vi "DecodeReplacement.vi"(1 "element":u8[](array[numeric]), 3 "Key":i32=-1, 5 "error in (no error)":errorcluster) -> (15 "element 2":u8[](array[numeric]), 16 "Replacement":T2(array[cluster]), 19 "error out":errorcluster)   [LabVIEW 2023, in "Referee.lvclass"]
uses:
  Referee.lvclass
panel:
  in  "Replacement 2":T1
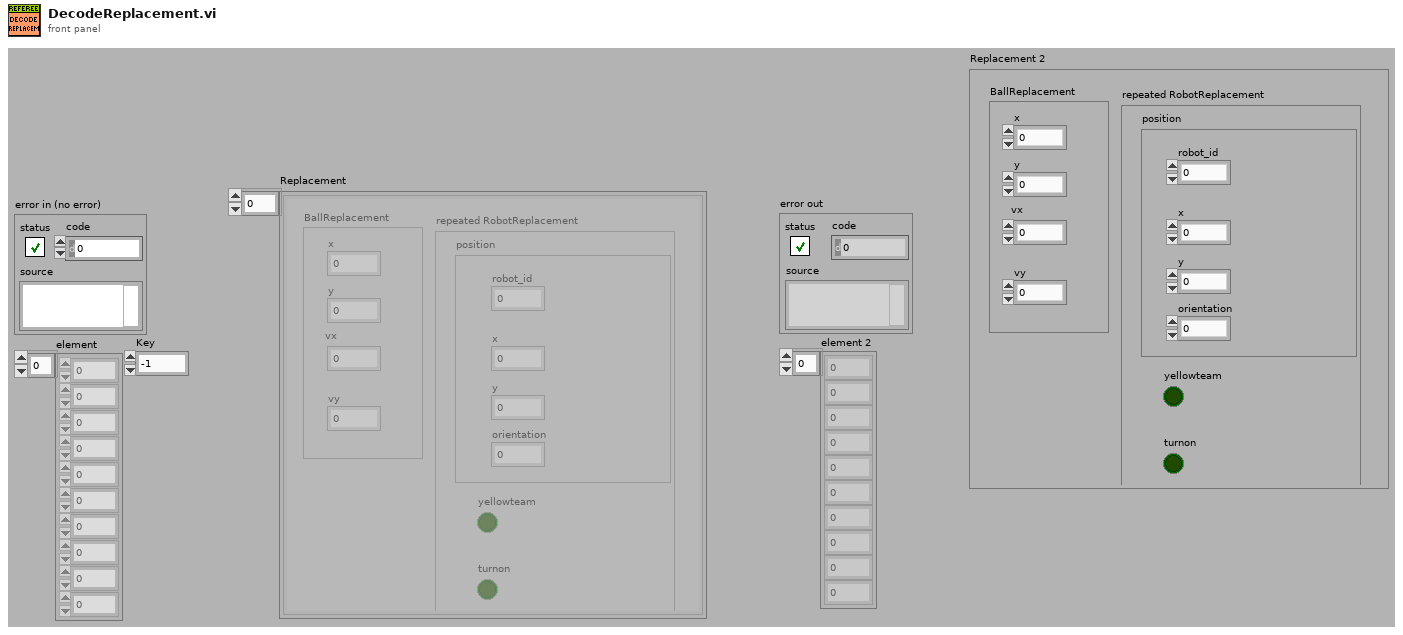
[diagram p1: front panel]
types:
  T1 = cluster{"BallReplacement":cluster{"x":dbl, "y":dbl, "vx":dbl, "vy":dbl}, "repeated RobotReplacement":cluster{"position":cluster{"robot_id":dbl, "x":dbl, "y":dbl, "orientation":dbl}, "yellowteam":bool, "turnon":bool}}
  T2 = cluster{"BallReplacement":cluster{"x":dbl, "y":dbl, "vx":dbl, "vy":dbl}, "repeated RobotReplacement":cluster{"position":cluster{"robot_id":dbl, "x":dbl, "y":dbl, "orientation":dbl}, "yellowteam":bool, "turnon":bool}}[]
  T3 = cluster{"position":cluster{"x\nx\nrobot_id":dbl, "x\nx\nx":dbl, "y":dbl, "orientation":dbl}, "yellowteam":bool, "turnon":bool}
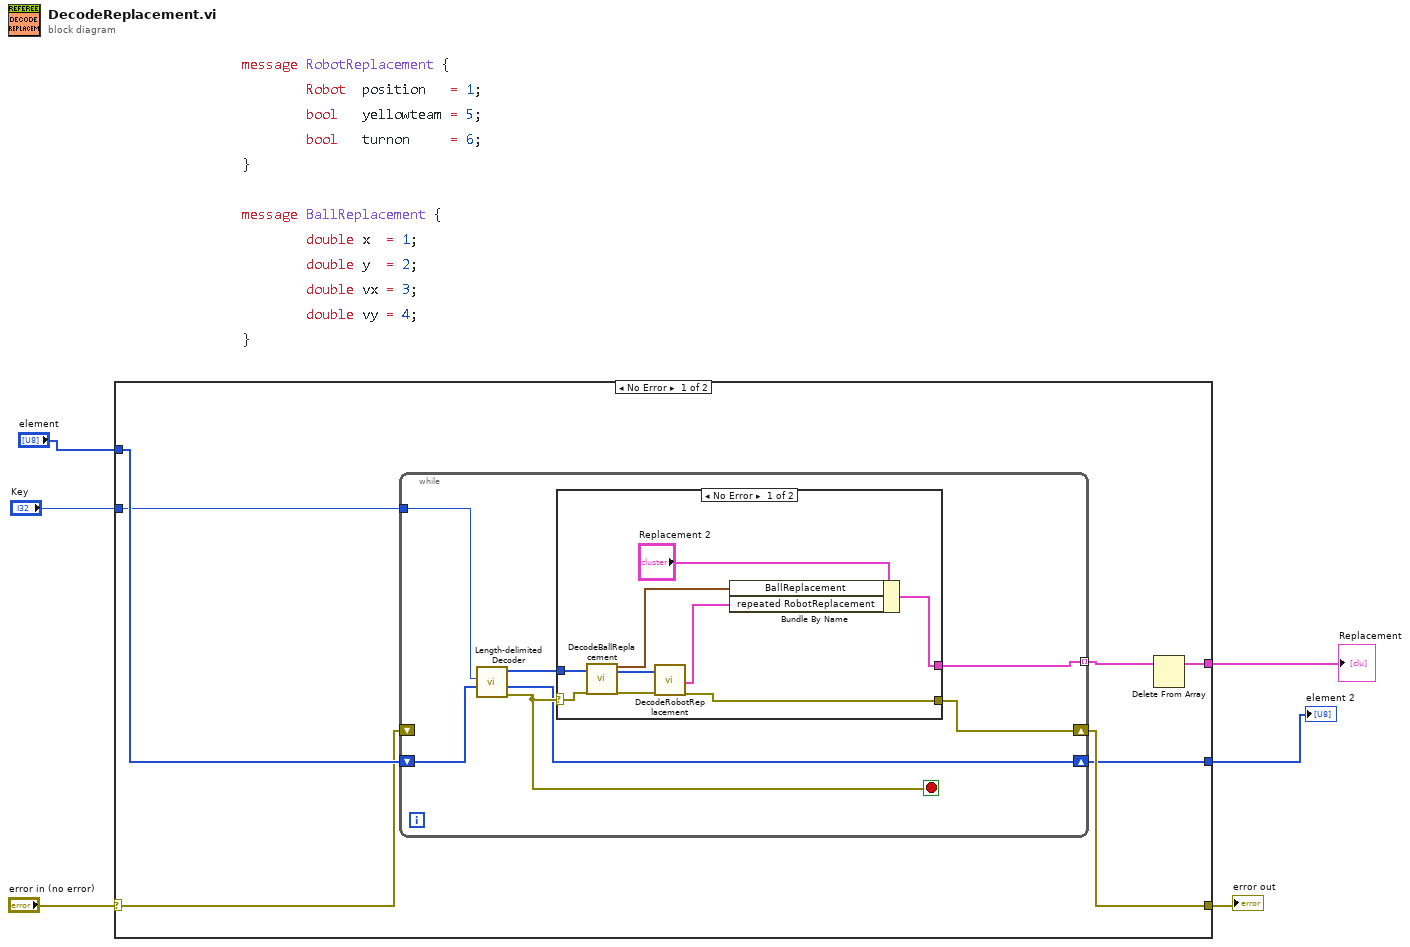
[diagram p0: block diagram]
diagram:
  n1 = case shown="No Error" "error in (no error)" {
    selector: "error in (no error)" -> [w10 w31]
    tunnel: [w9 w31] -> w5
    tunnel: "element" -> [w12 w30]
    tunnel: "Key" -> [w11 _]
    tunnel: [w8 _] -> w2
    tunnel: [w7 w30] -> w1
    frame No Error {
      n2 = while {
        tunnel: w11 -> [w18]
        shift-right: [w13] -> w7
        shift-left: w12 -> [w19]
        tunnel: [w17] -> w8 mode=indexing
        shift-right: [w15] -> w9
        shift-left: w10 -> [_]
        stop <- w16 stop-if-true
        n3 = call "Length-delimited Decoder.vi"("Array"=w19, "Key"=w18) -> ("error out"=w16:errorcluster, "array w/ subset deleted"=w13:u8[], "Length-delimited"=w14:u8[])  [unwired: 6 in, 1 out]
        n4 = case shown="No Error" w16 {
          selector: w16 -> [w26 w29]
          tunnel: w14 -> [w28 _]
          tunnel: [w23 _] -> w17
          tunnel: [w24 w29] -> w15
          frame No Error {
            n5 = call "DecodeBallReplacement.vi"("element"=w28, "error in (no error)"=w26) -> ("BallReplacement"=w21:cluster{"x":dbl, "y":dbl, "vx":dbl, "vy":dbl}, "element 2"=w27:u8[], "error out"=w25:errorcluster)  [unwired: 15 in]
            n6 = call "DecodeRobotReplacement.vi"("element"=w27, "error in (no error)"=w25) -> ("repeated RobotReplacement"=w20:T3, "error out"=w24:errorcluster)  [unwired: 15 in, 1 out]
            n7 = Bundle By Name(cluster="Replacement 2", "BallReplacement"=w21, "repeated RobotReplacement"=w20) -> (w23:T1)
          }
          frame Error {
          }
        }
      }
      n8 = Delete From Array(array=w8) -> ()  [unwired: 2 in, 2 out]
    }
    frame Error {
    }
  }
  "error out" <- w5
  "element 2" <- w1
  "Replacement" <- w2
